vi "updateTuplaEnDBImage.vi"(8 "error in":errorcluster, 11 "claseImagen in":refnum<class "claseImagen.lvclass">) -> (0 "error out":errorcluster, 3 "claseImagen out":refnum<class "claseImagen.lvclass">)   [LabVIEW 2014, in "claseImagen.lvclass"]
uses:
  claseImagen.lvclass
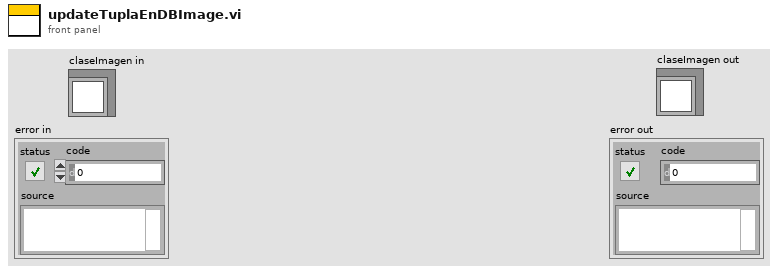
[diagram p1: front panel]
types:
  T1 = cluster{"idImage":dbl, "camposDeMedicionImage":string, "dateCreateImage":timestamp}
  T2 = cluster{dbl, "data":string, "ParaModificarAhoraHardcodeado":timestamp}
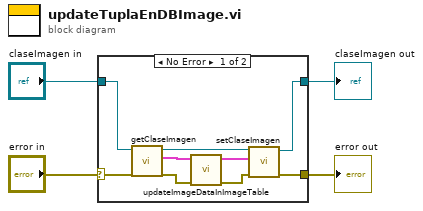
[diagram p0: block diagram]
diagram:
  n1 = case shown="No Error" "error in" {
    selector: "error in" -> [w11 w15]
    tunnel: [w10 w15] -> w3
    tunnel: [w12 w14] -> w2
    tunnel: "claseImagen in" -> [w13 w14]
    frame No Error {
      n2 = call "getClaseImagen.vi"("error in"=w11, "claseImagen in"=w13) -> ("error out"=w7:errorcluster, "dataReading"=w8:T1, "claseImagen out"=w9:refnum<class "claseImagen.lvclass">)  [unwired: 7 in]
      n3 = call "updateImageDataInImageTable.vi"("error in"=w7, "dataReadingToUpdate"=w8) -> ("error out"=w6:errorcluster, "dataUpdate"=w5:T2)  [unwired: 8 in]
      n4 = call "setClaseImagen.vi"("error in"=w6, "ImageDataIn"=w5, "claseImagen in"=w9) -> ("error out"=w10:errorcluster, "claseImagen out"=w12:refnum<class "claseImagen.lvclass">)  [unwired: 7 in]
    }
    frame Error {
    }
  }
  "claseImagen out" <- w2
  "error out" <- w3
